vi "Elevator Luncher.vi"   [LabVIEW 2022 SP3]
uses:
  Elevator Controller/Elevator Controller/Elevator Controller.lvclass
  C:/Program Files/National Instruments/LabVIEW 2022/vi.lib/ActorFramework/Actor/Actor.lvclass
  <vilib>/ActorFramework/Actor/Actor.lvclass
  C:/Workspace/CLA/Elevator AF_2022/Elevator Controller/Elevator Controller/Elevator Controller.lvclass
panel:
  # "Launcher"
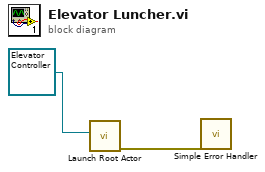
[diagram p0: block diagram]
diagram:
  n1 = call <vilib>:"Launch Root Actor.vi"("Actor"=refnum<class "Elevator Controller.lvclass"> refnum ("Elevator Controller.lvlib:Elevator Controller.lvclass")) -> ("error out"=w2:errorcluster)  [unwired: 9 in, 1 out]
  n2 = call <vilib>:"Simple Error Handler.vi"("error in (no error)"=w2) -> ()  [unwired: 4 in, 5 out]
